vi "Store LNA Queue.vi"(8 "error in (no error)":errorcluster, 9 "Message Enqueuer in":refnum<class "Message Enqueuer.lvclass">, 10 "Network Actor in":refnum<class "Client Proxy LNA.lvclass">, 11 "Server Controller in":refnum<class "Server Controller.lvclass">) -> (0 "error out":errorcluster, 3 "Server Controller out":refnum<class "Server Controller.lvclass">)   [LabVIEW 2016, in "Server Controller.lvlib" / "Server Controller.lvclass"]
uses:
  Server Controller.lvclass
  <vilib>/ActorFramework/Message Enqueuer/Message Enqueuer.lvclass
  Client Proxy LNA/Client Proxy LNA.lvclass
  Client Proxy LNA/Client Proxy LNA.lvclass/Client Proxy LNA.ctl
  Server Controller.lvclass/Server Controller.ctl
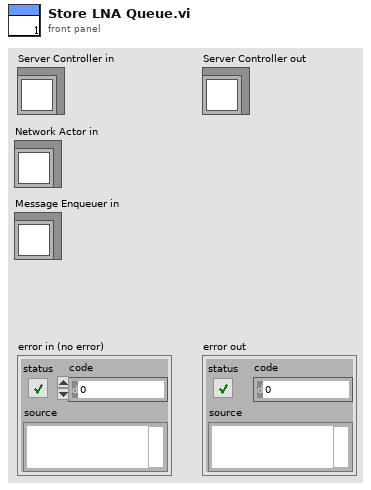
[diagram p1: front panel]
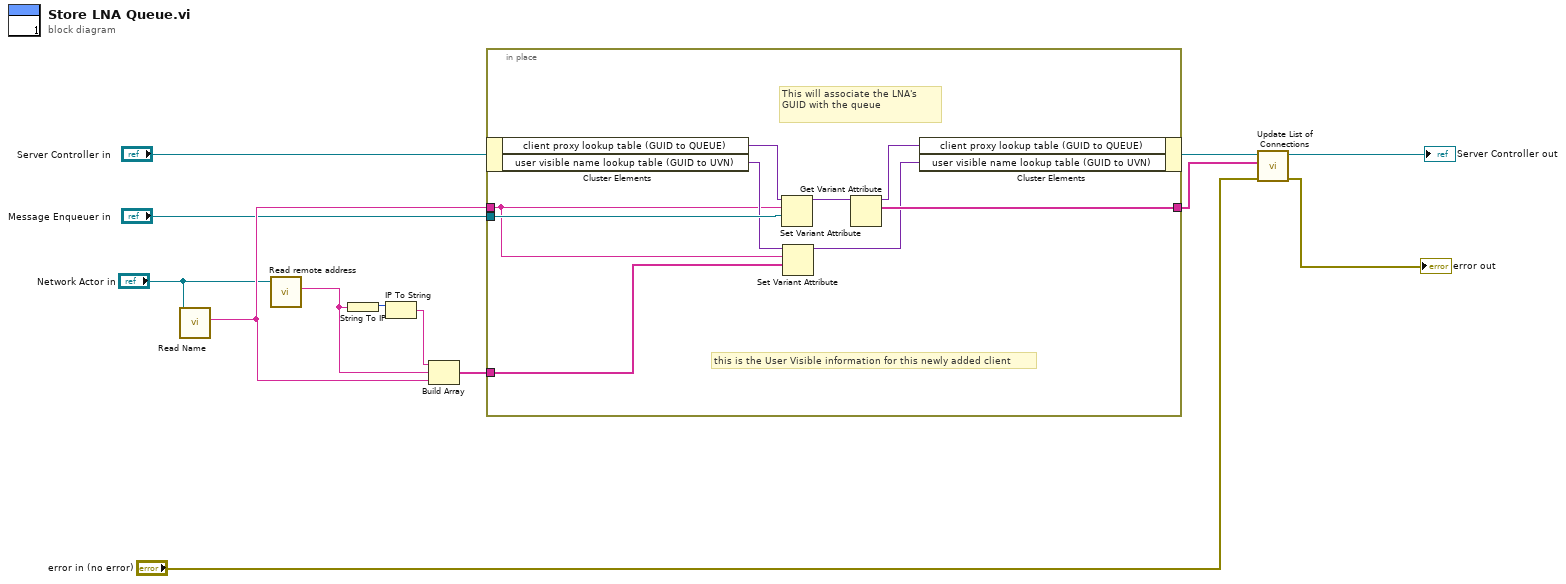
[diagram p0: block diagram]
diagram:
  n1 = call-dynamic "Read Name.vi"("Network Actor in"="Network Actor in") -> ("Name"=w6:string)  [unwired: 10 in]
  n2 = call "Read remote address.vi"("Client Proxy LNA in"="Network Actor in") -> ("remote address"=w10:string)  [unwired: 8 in, 2 out]
  n3 = String To IP(1:w10) -> (0:w9:u32)
  n4 = IP To String(2:w9) -> (0:w8:string)  [unwired: 1 in]
  n5 = Build Array(w8, w10, w6) -> (w2:string[])
  n6 = in-place {
    in-place-border: w6 -> [w15]
    in-place-border: "Message Enqueuer in" -> [w19]
    in-place-border: [w18] -> w4
    in-place-border: w2 -> [w14]
    # "this is the User Visible information for this newly added client"
    # "This will associate the LNA's GUID with the queue"
    n7 = in-place-cluster #1("Server Controller in") -> ("client proxy lookup table (GUID to QUEUE)"=w22:variant, "user visible name lookup table (GUID to UVN)"=w17:variant)
    n8 = Set Variant Attribute(Variant=w22, name=w15, value=w19) -> (Variant out=w21:variant)  [unwired: 1 in, 2 out]
    n9 = Set Variant Attribute(Variant=w17, name=w15, value=w14) -> (Variant out=w16:variant)  [unwired: 1 in, 2 out]
    n10 = Get Variant Attribute(Variant=w21) -> (duplicate Variant=w20:variant, names=w18:string[])  [unwired: 3 in, 2 out]
    n11 = in-place-cluster #1("client proxy lookup table (GUID to QUEUE)"=w20, "user visible name lookup table (GUID to UVN)"=w16) -> (w3:refnum<class "Server Controller.lvclass">)
  }
  n12 = call "Update List of Connections.vi"("error in (no error)"="error in (no error)", "GUIDs"=w4, "Server Controller in"=w3) -> ("error out"=→"error out":errorcluster, "Server Controller out"=→"Server Controller out":refnum<class "Server Controller.lvclass">)  [unwired: 7 in]
